vi "Init.vi"(8 "error in (no error)":errorcluster) -> (0 "error out":errorcluster, 3 "FormulaLV App out":refnum<class "FormulaG App.lvclass">)   [LabVIEW 2020, in "FormulaG.lvlib" / "FormulaG App.lvclass"]
uses:
  FormulaG App.lvclass
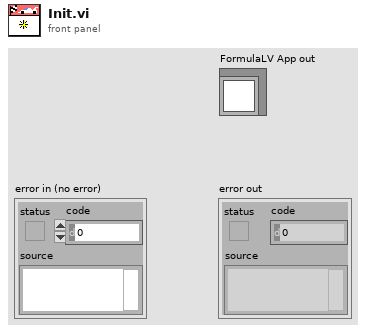
[diagram p1: front panel]
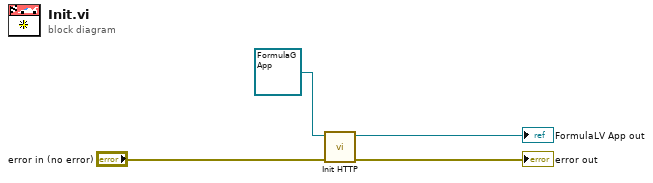
[diagram p0: block diagram]
diagram:
  n1 = call "Init HTTP.vi"("error in (no error)"="error in (no error)", "FormulaLV App in"=refnum<class "FormulaG App.lvclass"> refnum) -> ("error out"=→"error out":errorcluster, "FormulaLV App out"=→"FormulaLV App out":refnum<class "FormulaG App.lvclass">)  [unwired: 8 in]
